vi "Untitled 7 (SubVI).vi"(11 "Path":path) -> (2 "Session Generator Output":string)   [LabVIEW 2015]
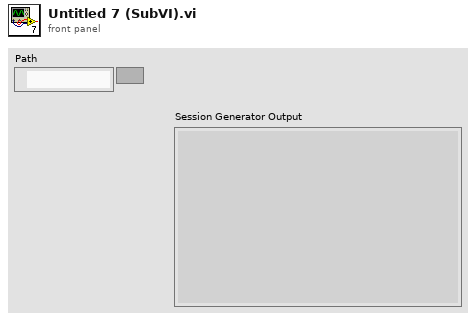
[diagram p1: front panel]
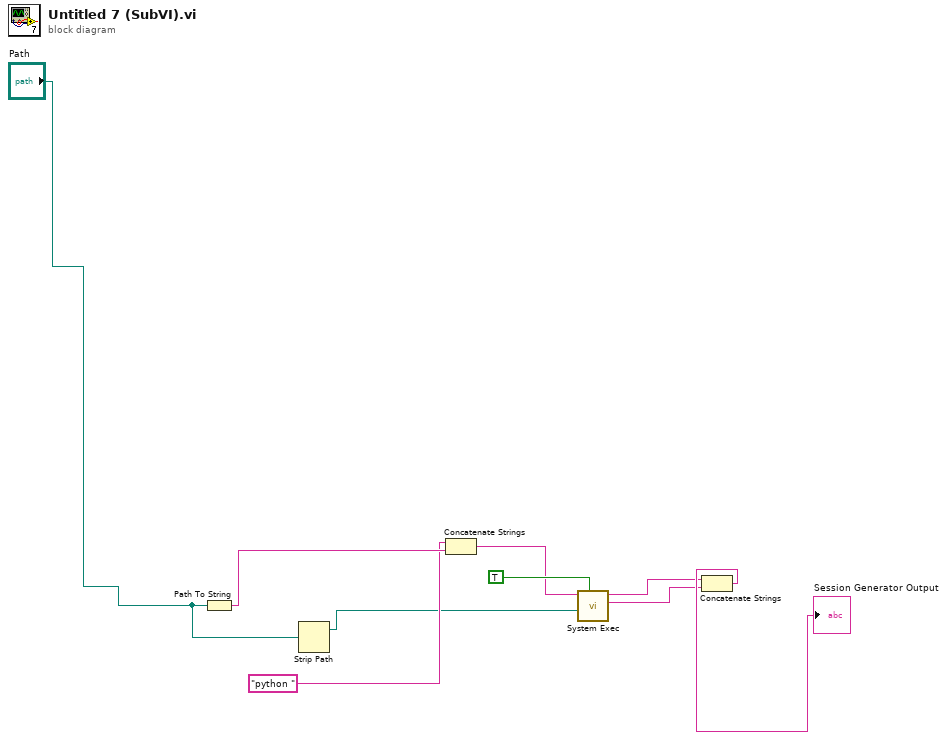
[diagram p0: block diagram]
diagram:
  w7 = TRUE
  n1 = Path To String(path="Path") -> (string=w6:string)
  n2 = Strip Path(path="Path") -> (stripped path=w1:path)  [unwired: 1 out]
  n3 = Concatenate Strings("python ", w6) -> (w5:string)
  n4 = call <vilib>:"System Exec.vi"("run minimized? (F)"=w7, "wait until completion? (T)"=w7, "working directory"=w1, "command line"=w5) -> ("standard error"=w3:string, "standard output"=w4:string)  [unwired: 4 in, 2 out]
  n5 = Concatenate Strings(w4, w3) -> (→"Session Generator Output":string)
